vi "temp sweep(SubVI).vi"(0 "data":refnum<queue>, 5 "steps number":i32, 7 "ch str":string, 9 "Temperature":dbl=300.0, 11 "config":refnum<queue>, 12 "Instrument Ref":refnum<k24>, 13 "Temperature 2":dbl=300.0, 14 "Rate":dbl=10.0) -> (8 "错误输出":errorcluster)   [LabVIEW 2019, in "SubVI.lvlib"]
uses:
  SubVI.lvlib
  lib/QDInstrument.dll
  config.ctl
panel:
  out "Temperature\nStatus":i32(ring) items=["TemperatureUnknown"=0, "Stable"=1, "Tracking"=2, "Near"=5, "Chasing"=6, "Filling"=7, "Standby"=10, "Disabled"=13, "ImpedanceNotFunction"=14, "TempFailure"=15]
  # "(真是通道1，假是通道2)"
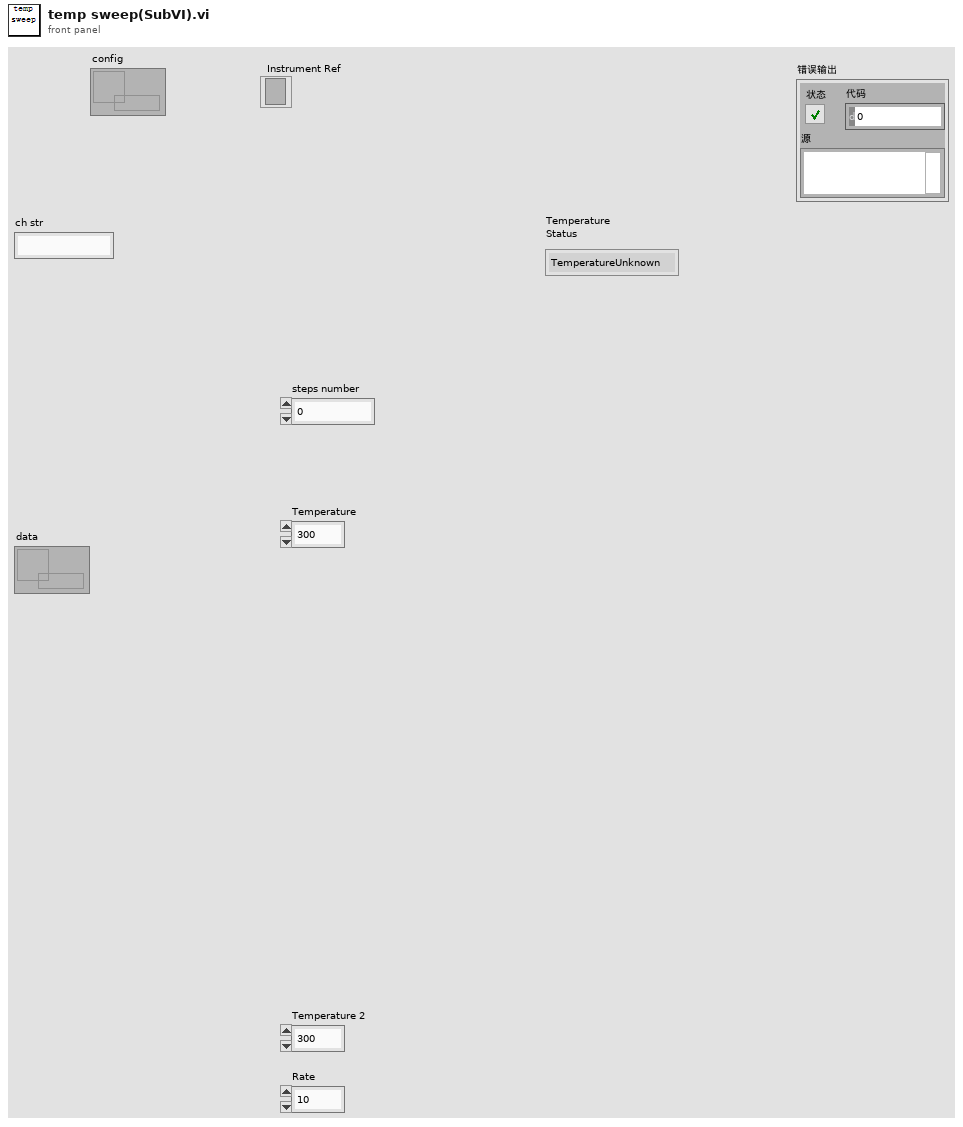
[diagram p1: front panel]
types:
  T1 = typedef "config.ctl" = cluster{"error":bool, "initialize":string, "数值":dbl, "6221":cluster{"6221 Resource":refnum<visa-resource-name>, "Delta status":bool}, "7001":cluster{"Ch":bool}}
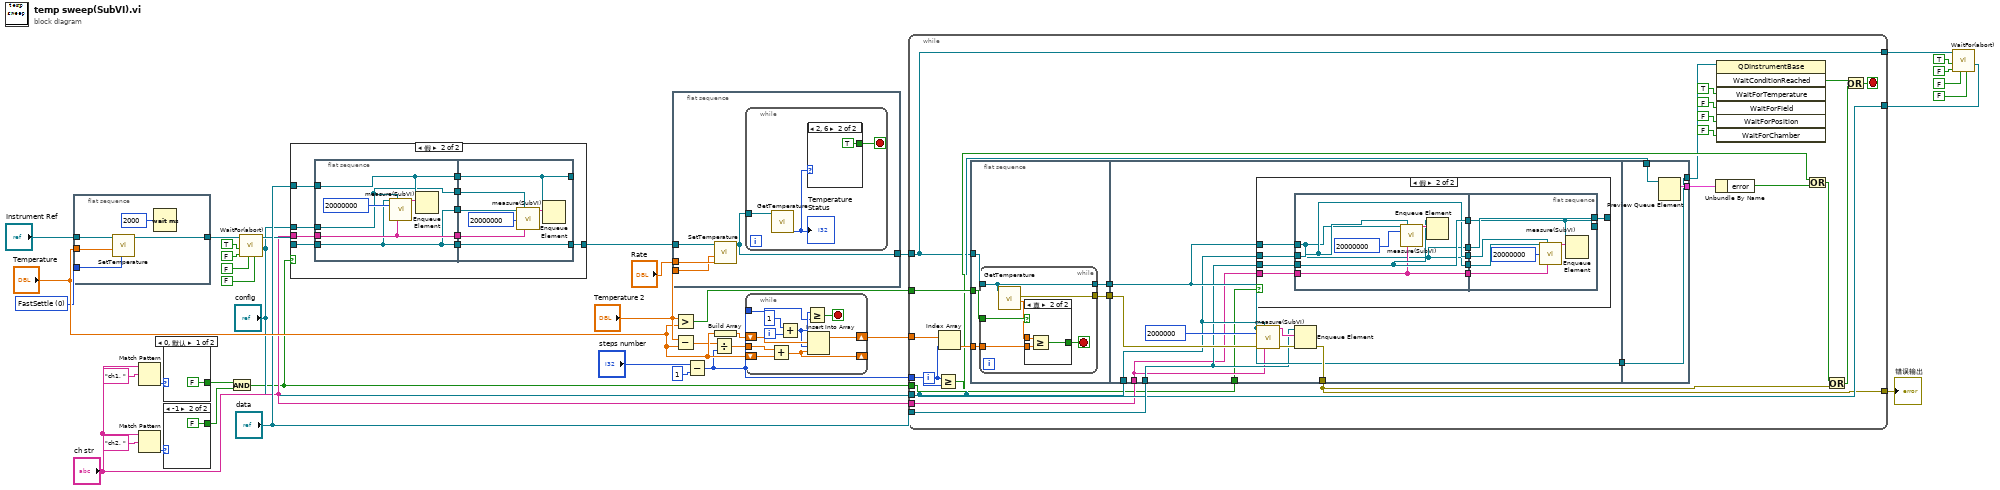
[diagram p0: block diagram]
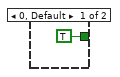
[diagram p2: hidden frame]
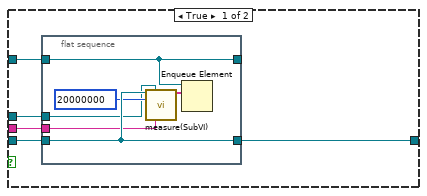
[diagram p3: hidden frame]
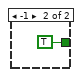
[diagram p4: hidden frame]
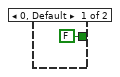
[diagram p5: hidden frame]
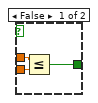
[diagram p6: hidden frame]
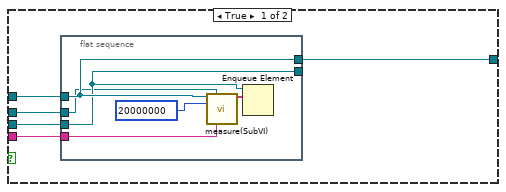
[diagram p7: hidden frame]
diagram:
  w25 = 0 items=["FastSettle", "NoOvershoot"] ("Approach")
  n1 = flat-sequence {
    tunnel: "Temperature" -> [w43]
    tunnel: [w42] -> w30
    tunnel: w25 -> [w41]
    tunnel: "Instrument Ref" -> [w40]
    frame #0 {
      n2 = call "SetTemperature.vi"("Approach"=w41, "Temperature"=w43, "Instrument Ref In"=w40) -> ("Instrument Ref Out"=w42:refnum<k24>)  [unwired: 4 in, 2 out]
      n3 = Wait (ms)(milliseconds to wait=u32 2000) -> ()  [unwired: 1 out]
    }
  }
  n4 = Match Pattern(string="ch str", regular expression="ch1, " ("正则表达式")) -> (offset past match=w10:i32)  [unwired: 1 in, 3 out]
  n5 = Match Pattern(string="ch str", regular expression="ch2, " ("正则表达式")) -> (offset past match=w9:i32)  [unwired: 1 in, 3 out]
  n6 = case shown="0, 默认" w10 {
    tunnel: [FALSE TRUE] -> w8
    frame 0, Default {
    }
    frame -1 {
    }
  }
  n7 = case shown="-1" w9 {
    tunnel: [TRUE FALSE] -> w7
    frame 0, Default {
    }
    frame -1 {
    }
  }
  n8 = And(x=w8, y=w7) -> (x .and. y?=w1:bool)
  n9 = call "WaitFor(abort).vi"("config"="config", "Wait For Chamber"=FALSE, "Wait For Position"=FALSE, "Wait For Field"=FALSE, "Wait For Temperature"=TRUE, "Instrument Ref In"=w30) -> ("Instrument Ref Out"=w5:refnum<k24>)  [unwired: 4 in, 1 out]
  n10 = case shown="假" w1 {
    tunnel: w5 -> [w52 w68]
    tunnel: "ch str" -> [w51 w67]
    tunnel: "data" -> [w50 w66]
    tunnel: "config" -> [w49 w65]
    tunnel: [w48 w64] -> w4
    frame True {
      n11 = flat-sequence {
        tunnel: w52 -> [w58]
        tunnel: [w58] -> w48
        tunnel: w51 -> [w56]
        tunnel: [w54] -> _
        tunnel: w50 -> [w54]
        tunnel: w49 -> [w53]
        frame #0 {
          n12 = call "measure(SubVI).vi"(".NET引用句柄输入"=w58, "config"=w53, "Timeout (20000 ms)"=u32 20000000, "ch str"=w56) -> ("data"=w55:string[])  [unwired: 10 in, 1 out]
          n13 = Enqueue Element(queue=w54, element=w55) -> ()  [unwired: 2 in, 3 out]
        }
      }
    }
    frame False {
      n14 = flat-sequence {
        tunnel: w68 -> [w69]
        tunnel: w67 -> [w70]
        tunnel: w66 -> [w72]
        tunnel: w65 -> [w71]
        tunnel: [w69] -> w63
        tunnel: [w72] -> w62
        tunnel: [w71] -> w61
        tunnel: [w70] -> w60
        tunnel: [w69] -> w59
        tunnel: [w75] -> _
        tunnel: [w81] -> w64
        tunnel: w63 -> [w81]
        tunnel: w62 -> [w75]
        tunnel: w61 -> [w78]
        tunnel: w60 -> [w77]
        tunnel: w59 -> [w76]
        frame #0 {
          n15 = call "measure(SubVI).vi"(".NET引用句柄输入"=w69, "config"=w71, "Timeout (20000 ms)"=u32 20000000, "ch str"=w70) -> ("data"=w73:string[])  [unwired: 10 in, 1 out]
          n16 = Enqueue Element(queue=w72, element=w73) -> ()  [unwired: 2 in, 3 out]
        }
        frame #1 {
          n17 = call "measure(SubVI).vi"(".NET引用句柄输入"=w76, "config"=w78, "Timeout (20000 ms)"=u32 20000000, "ch str"=w77) -> ("data"=w80:string[])  [unwired: 10 in, 1 out]
          n18 = Enqueue Element(queue=w75, element=w80) -> ()  [unwired: 2 in, 3 out]
        }
      }
    }
  }
  n19 = flat-sequence {
    tunnel: "Temperature 2" -> [w84]
    tunnel: [w82] -> w34
    tunnel: w4 -> [w83]
    tunnel: "Rate" -> [w85]
    frame #0 {
      n20 = call "SetTemperature.vi"("Rate"=w85, "Temperature"=w84, "Instrument Ref In"=w83) -> ("Instrument Ref Out"=w82:refnum<k24>)  [unwired: 4 in, 2 out]
      n21 = while {
        tunnel: w82 -> [w86]
        stop <- w87 stop-if-true
        n22 = call "GetTemperature.vi"("Instrument Ref In"=w86) -> ("Temperature\nStatus"=w88:i32)  [unwired: 4 in, 4 out]
        "Temperature\nStatus" <- w88
        n23 = case shown="2, 6" w88 {
          tunnel: [FALSE TRUE] -> w87
          frame 0, Default {
          }
          frame 2, 6 {
          }
        }
      }
    }
  }
  n24 = Greater?(x="Temperature 2", y="Temperature") -> (0:w37:bool)
  n25 = Subtract(x="Temperature 2", y="Temperature") -> (x-y=w33:dbl)
  n26 = Subtract(x="steps number", y=1) -> (x-y=w14:i32)
  n27 = Divide(x=w33, y=w14) -> (x/y=w31:dbl)
  n28 = Build Array("Temperature") -> (w32:dbl[])
  n29 = while {
    shift-right: [w100] -> w38
    shift-left: w32 -> [w99]
    tunnel: w31 -> [w94]
    tunnel: w14 -> [w93]
    shift-right: [w92] -> _
    shift-left: "Temperature" -> [w91]
    i -> [w98]
    stop <- w95 stop-if-true
    n30 = Add(x=w94, y=w91) -> (x+y=w92:dbl)
    n31 = Add(x=1, y=w98) -> (x+y=w96:i32)
    n32 = Greater Or Equal?(x=w96, y=w93) -> (x >= y?=w95:bool)
    n33 = Insert Into Array(array=w99, index=w96, new element=w92) -> (w100:dbl[])
  }
  n34 = while {
    tunnel: w34 -> [w111]
    tunnel: w37 -> [w126]
    tunnel: w38 -> [w125]
    tunnel: w14 -> [w120]
    tunnel: "data" -> [w122]
    tunnel: "config" -> [w118]
    tunnel: [w111] -> w20
    tunnel: [w118] -> w18
    tunnel: [w105] -> w17
    tunnel: "ch str" -> [w104]
    tunnel: w1 -> [w101]
    i -> [w119]
    stop <- w108 stop-if-true
    n35 = Greater Or Equal?(x=w119, y=w120) -> (x >= y?=w121:bool)
    n36 = Index Array(array=w125, index=w119) -> (element=w124:dbl)
    n37 = flat-sequence {
      tunnel: w111 -> [w131]
      tunnel: w126 -> [w130]
      tunnel: w124 -> [w129]
      tunnel: [w128] -> w123
      tunnel: [w127] -> w117
      tunnel: w123 -> [w148]
      tunnel: w122 -> [w146]
      tunnel: w118 -> [w147]
      tunnel: [w150] -> w105
      tunnel: w117 -> [w152]
      tunnel: [w148] -> w106
      tunnel: w104 -> [w145]
      tunnel: w101 -> [w144]
      tunnel: w118 -> [w190]
      tunnel: [w189] -> w103
      tunnel: [w188] -> w107
      tunnel: w106 -> [w188]
      frame #0 {
        n38 = while {
          tunnel: w131 -> [w133]
          tunnel: w130 -> [w137]
          tunnel: w129 -> [w135]
          tunnel: [w133] -> w128
          tunnel: [w132] -> w127
          stop <- w134 stop-if-true
          n39 = call "GetTemperature.vi"("Instrument Ref In"=w133) -> ("Temperature"=w136:dbl, "error out"=w132:errorcluster)  [unwired: 4 in, 3 out]
          n40 = case shown="真" w137 {
            tunnel: w136 -> [w140 w143]
            tunnel: w135 -> [w139 w142]
            tunnel: [w138 w141] -> w134
            frame False {
              n41 = Less Or Equal?(x=w140, y=w139) -> (x <= y?=w138:bool)
            }
            frame True {
              n42 = Greater Or Equal?(x=w143, y=w142) -> (x >= y?=w141:bool)
            }
          }
        }
      }
      frame #1 {
        n43 = case shown="假" w144 {
          tunnel: w148 -> [w158 w174]
          tunnel: w145 -> [w157 w173]
          tunnel: w146 -> [w156 w172]
          tunnel: w147 -> [w155 w171]
          tunnel: [w154 w170] -> _
          frame True {
            n44 = flat-sequence {
              tunnel: w158 -> [w164]
              tunnel: [w164] -> w154
              tunnel: w157 -> [w162]
              tunnel: [w160] -> _
              tunnel: w156 -> [w160]
              tunnel: w155 -> [w159]
              frame #0 {
                n45 = call "measure(SubVI).vi"(".NET引用句柄输入"=w164, "config"=w159, "Timeout (20000 ms)"=u32 20000000, "ch str"=w162) -> ("data"=w161:string[])  [unwired: 10 in, 1 out]
                n46 = Enqueue Element(queue=w160, element=w161) -> ()  [unwired: 2 in, 3 out]
              }
            }
          }
          frame False {
            n47 = flat-sequence {
              tunnel: w174 -> [w175]
              tunnel: w173 -> [w176]
              tunnel: w172 -> [w178]
              tunnel: w171 -> [w177]
              tunnel: [w175] -> w169
              tunnel: [w178] -> w168
              tunnel: [w177] -> w167
              tunnel: [w176] -> w166
              tunnel: [w175] -> w165
              tunnel: [w181] -> _
              tunnel: [w187] -> w170
              tunnel: w169 -> [w187]
              tunnel: w168 -> [w181]
              tunnel: w167 -> [w184]
              tunnel: w166 -> [w183]
              tunnel: w165 -> [w182]
              frame #0 {
                n48 = call "measure(SubVI).vi"(".NET引用句柄输入"=w175, "config"=w177, "Timeout (20000 ms)"=u32 20000000, "ch str"=w176) -> ("data"=w179:string[])  [unwired: 10 in, 1 out]
                n49 = Enqueue Element(queue=w178, element=w179) -> ()  [unwired: 2 in, 3 out]
              }
              frame #1 {
                n50 = call "measure(SubVI).vi"(".NET引用句柄输入"=w182, "config"=w184, "Timeout (20000 ms)"=u32 20000000, "ch str"=w183) -> ("data"=w186:string[])  [unwired: 10 in, 1 out]
                n51 = Enqueue Element(queue=w181, element=w186) -> ()  [unwired: 2 in, 3 out]
              }
            }
          }
        }
        n52 = call "measure(SubVI).vi"(".NET引用句柄输入"=w148, "config"=w147, "Timeout (20000 ms)"=u32 2000000, "error in (no error)"=w152, "ch str"=w145) -> ("data"=w153:string[], "error out"=w151:errorcluster)  [unwired: 9 in]
        n53 = Enqueue Element(queue=w146, element=w153, error in (no error)=w151) -> (error out=w150:errorcluster)  [unwired: 1 in, 2 out]
      }
      frame #2 {
        n54 = Preview Queue Element(queue=w190) -> (element=w189:T1)  [unwired: 2 in, 3 out]
      }
    }
    n55 = Unbundle By Name(w103) -> ("error"=w102:bool)
    n56 = invoke class="QDInstrumentBase" method="WaitConditionReached"(reference=w107, "WaitForTemperature"=TRUE, "WaitForField"=FALSE, "WaitForPosition"=FALSE, "WaitForChamber"=FALSE) -> ("WaitConditionReached"=w110:bool)  [unwired: 2 in, 6 out]
    n57 = Or(x=w121, y=w102) -> (x .or. y?=w116:bool)
    n58 = Or(x=w116, y=w105) -> (x .or. y?=w109:bool)
    n59 = Or(x=w110, y=w109) -> (x .or. y?=w108:bool)
  }
  "错误输出" <- w17
  n60 = call "WaitFor(abort).vi"("config"=w18, "Wait For Chamber"=FALSE, "Wait For Position"=FALSE, "Wait For Field"=FALSE, "Wait For Temperature"=TRUE, "Instrument Ref In"=w20) -> ()  [unwired: 4 in, 2 out]
